vi "NI_6501_DIO.vi"() -> ()   [LabVIEW 2024]
uses:
  <vilib>/DAQmx/read.llb/DAQmx Read (Digital Bool 1Line 1Point).vi
  <vilib>/DAQmx/write.llb/DAQmx Write (Digital Bool 1Line 1Point).vi
  <vilib>/DAQmx/create/channels.llb/DAQmx Create Channel (DI-Digital Input).vi
  <vilib>/DAQmx/miscellaneous.llb/DAQmx Fill In Error Info.vi
  <vilib>/DAQmx/create/channels.llb/DAQmx Create Channel (DO-Digital Output).vi
panel:
  in  "lines 2":tag
  out "data":bool
  in  "选择输出或输入":bool
  in  "输出":bool
  in  "line grouping":i32(ring)=1 items=["one channel for each line", "one channel for all lines"]
  in  "lines":tag
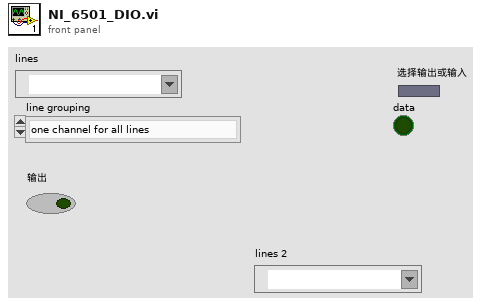
[diagram p1: front panel]
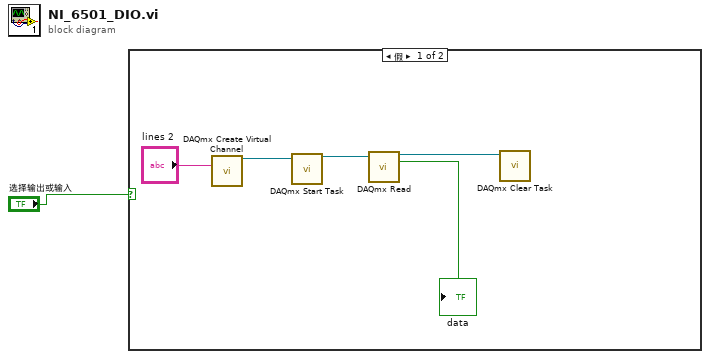
[diagram p0: block diagram]
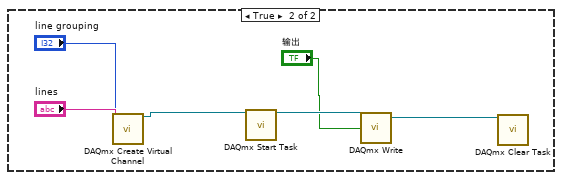
[diagram p2: hidden frame]
diagram:
  n1 = case shown="假" "选择输出或输入" {
    frame False {
      n2 = call-poly <vilib>:"DAQmx Create Virtual Channel.vi"("lines"="lines 2") -> ("task out"=w6:refnum<k21>)  [unwired: 13 in, 1 out]
      n3 = call <vilib>:"DAQmx Start Task.vi"("task/channels in"=w6) -> ("task out"=w5:refnum<k21>)  [unwired: 13 in, 1 out]
      n4 = call-poly <vilib>:"DAQmx Read.vi"("task/channels in"=w5) -> ("task out"=w4:refnum<k21>, "data"=→"data":bool)  [unwired: 12 in, 1 out]
      n5 = call <vilib>:"DAQmx Clear Task.vi"("task in"=w4) -> ()  [unwired: 14 in, 1 out]
    }
    frame True {
      n6 = call-poly <vilib>:"DAQmx Create Virtual Channel.vi"("lines"="lines", "line grouping"="line grouping") -> ("task out"=w10:refnum<k21>)  [unwired: 12 in, 1 out]
      n7 = call <vilib>:"DAQmx Start Task.vi"("task/channels in"=w10) -> ("task out"=w9:refnum<k21>)  [unwired: 13 in, 1 out]
      n8 = call-poly <vilib>:"DAQmx Write.vi"("task/channels in"=w9, "data"="输出") -> ("task out"=w8:refnum<k21>)  [unwired: 11 in, 2 out]
      n9 = call <vilib>:"DAQmx Clear Task.vi"("task in"=w8) -> ()  [unwired: 14 in, 1 out]
    }
  }
